vi "Next Code Point.vi"(10 "Index":i32=-1, 11 "Tokenizer In":T1) -> (3 "Tokenizer":T1)   [LabVIEW 2020, in "Stream.lvlib" / "URLPattern.lvclass"]
uses:
  URLPattern.lvclass
  Tokenizer.ctl
  Tokenize Policy.ctl
  Token.ctl
  Token Type.ctl
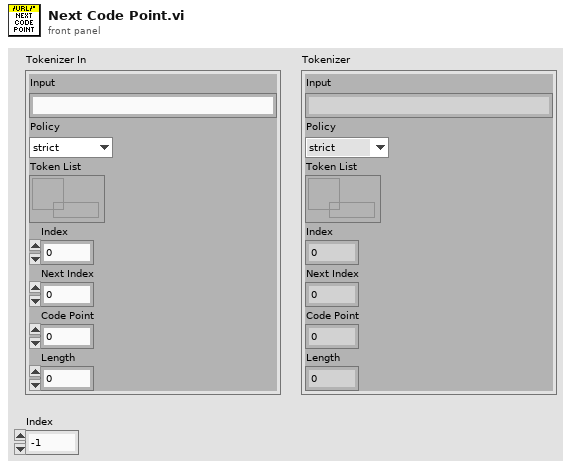
[diagram p1: front panel]
types:
  T1 = typedef "Stream.lvlib/URLPattern.lvclass/Tokenizer.ctl" = cluster{"Input":string, "Policy":T2, "Token List":refnum<queue>, "Index":i32, "Next Index":i32, "Code Point":u32, "Length":i32}
  T2 = typedef "Stream.lvlib/URLPattern.lvclass/Tokenize Policy.ctl" = enum16{"strict", "lenient"}
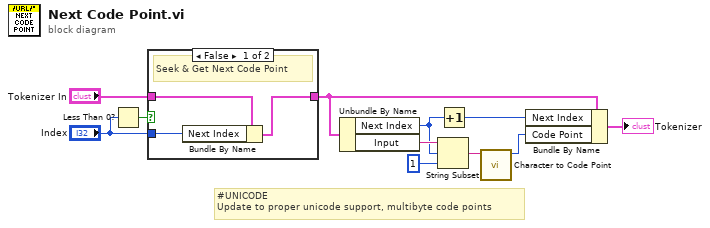
[diagram p0: block diagram]
diagram:
  # "#UNICODE\nUpdate to proper unicode support, multibyte code points"
  n1 = Less Than 0?(x="Index") -> (x < 0?=w3:bool)
  n2 = case shown="False" w3 {
    tunnel: "Tokenizer In" -> [w14 w15]
    tunnel: "Index" -> [w12 _]
    tunnel: [w13 w15] -> w2
    frame False {
      # "Seek & Get Next Code Point"
      n3 = Bundle By Name(cluster=w14, "Next Index"=w12) -> (w13:T1)
    }
    frame True {
      # "Get Next Code Point"
    }
  }
  n4 = Unbundle By Name(w2) -> ("Next Index"=w1:i32, "Input"=w8:string)
  n5 = String Subset(string=w8, offset (0)=w1, length (rest)=1 ("length (rest)")) -> (substring=w10:string)
  n6 = Increment(x=w1) -> (x+1=w9:i32)
  n7 = call "Character to Code Point.vi"("Character"=w10) -> ("U32 Code Point"=w7:u32)  [unwired: 9 in, 1 out]
  n8 = Bundle By Name(cluster=w2, "Next Index"=w9, "Code Point"=w7) -> (→"Tokenizer":T1)
